vi "GetPosition.vi"(4 "error in (no error)":errorcluster, 5 "Motor":i32, 6 "DeviceKey In":string, 7 "CmdLib In":refnum<k24>) -> (0 "error out":errorcluster, 1 "Position":i32, 2 "DeviceKey Out":string, 3 "CmdLib Out":refnum<k24>)   [LabVIEW 2014]
uses:
  C:/Users/Hexagon/Documents/git/DevPyController/labview/cesium_controller/PicoMotor/NewFocus8742/CmdLib.dll
  CmdLib.dll
panel:
  in  "pos":i32
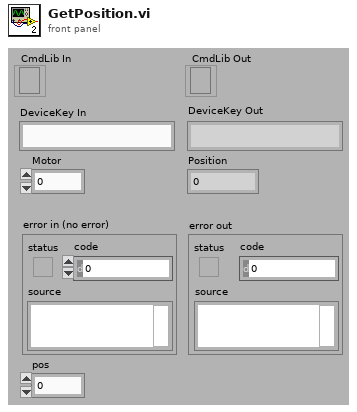
[diagram p1: front panel]
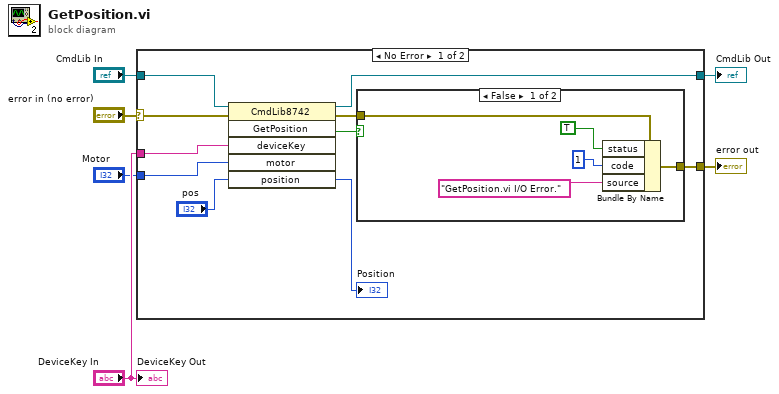
[diagram p0: block diagram]
diagram:
  n1 = case shown="No Error" "error in (no error)" {
    selector: "error in (no error)" -> [w12 w23]
    tunnel: "CmdLib In" -> [w16 w24]
    tunnel: [w15 w24] -> w5
    tunnel: "Motor" -> [w14 _]
    tunnel: "DeviceKey In" -> [w13 _]
    tunnel: [w9 w23] -> w2
    frame No Error {
      n2 = invoke class="CmdLib8742" method="GetPosition"(reference=w16, error in=w12, "deviceKey"=w13, "motor"=w14, "position"="pos") -> (reference out=w15:refnum<k24>, error out=w10:errorcluster, "GetPosition"=w11:bool, "position"=→"Position":i32)  [unwired: 1 in, 2 out]
      n3 = case shown="False" w11 {
        tunnel: w10 -> [w21 w22]
        tunnel: [w20 w22] -> w9
        frame False {
          n4 = Bundle By Name(cluster=w21, "status"=TRUE, "code"=1, "source"="GetPosition.vi I/O Error.") -> (w20:errorcluster)
        }
        frame True {
        }
      }
    }
    frame Error {
    }
  }
  "error out" <- w2
  "CmdLib Out" <- w5
  "DeviceKey Out" <- "DeviceKey In"
